vi "I2C Timestamp Loop.vi"(0 "fpga interface in":refnum<k20>, 1 "'stop' notifier":refnum<notifier>, 2 "log i2c to disk":bool=TRUE, 5 "tdms file directory":path, 9 "timestamp filter":T1[](array[typedef])=[enum."User24", enum."User25", enum."User26", enum."User27", enum."User28", enum."User29", enum."User30", enum."User31"], 11 "error in (no error)":errorcluster) -> (4 "i2c data":string[][](array[string]), 15 "error out":errorcluster)   [LabVIEW 2023, in "GettingStarted_Common_148X_Host.lvlib"]
uses:
  GettingStarted_Common_148X_Host.lvlib
  <instrlib>/FlexRIO/CSI-2/v2/FPGA/Types/Timestamp ID.ctl
  <instrlib>/FlexRIO/CSI-2/v2/FPGA/NI CSI-2 API FPGA v2.lvlib
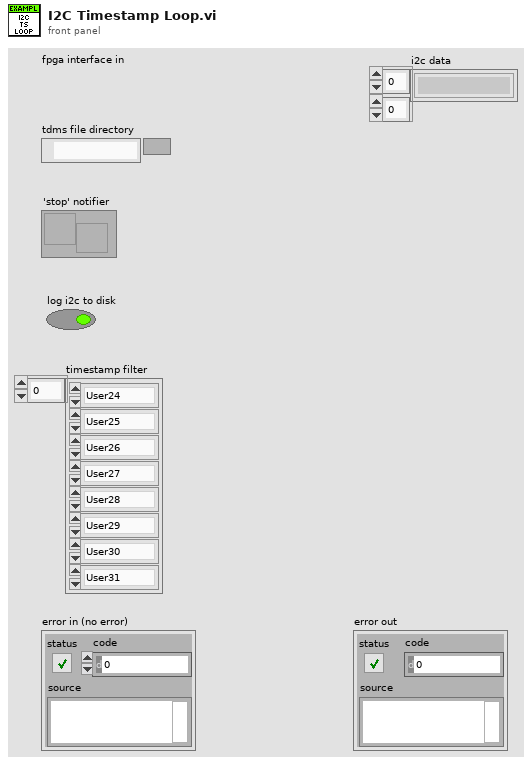
[diagram p1: front panel]
types:
  T1 = typedef "NI CSI-2 API FPGA v2.lvlib/Timestamp ID.ctl" = enum8{"SI0 LLP", "SI1 LLP", "SI2 LLP", "SI3 LLP", "SI4 LLP", "SI5 LLP", "SI6 LLP", "SI7 LLP", "SO0 LLP", "SO1 LLP", "SO2 LLP", "SO3 LLP", "SO4 LLP", "SO5 LLP", "SO6 LLP", "SO7 LLP", "Ser0 GPIO Bank", "Ser1 GPIO Bank", "Ser2 GPIO Bank", "Ser3 GPIO Bank", "Ser4 GPIO Bank", "Ser5 GPIO Bank", "Ser6 GPIO Bank", "Ser7 GPIO Bank", "Des0 GPIO Bank", "Des1 GPIO Bank", "Des2 GPIO Bank", "Des3 GPIO Bank", "Des4 GPIO Bank", "Des5 GPIO Bank", "Des6 GPIO Bank", "Des7 GPIO Bank", "User0", "User1", "User2", "User3", "User4", "User5", "User6", "User7", "User8", "User9", "User10", "User11", "User12", "User13", "User14", "User15", "User16", "User17", "User18", "User19", "User20", "User21", "User22", "User23", "User24", "User25", "User26", "User27", "User28", "User29", "User30", "User31"}
  T2 = typedef "NI CSI-2 API FPGA v2.lvlib/User Timestamp.ctl" = cluster{"valid":bool, "user data":fxp<+,58,58>, "id":T1}
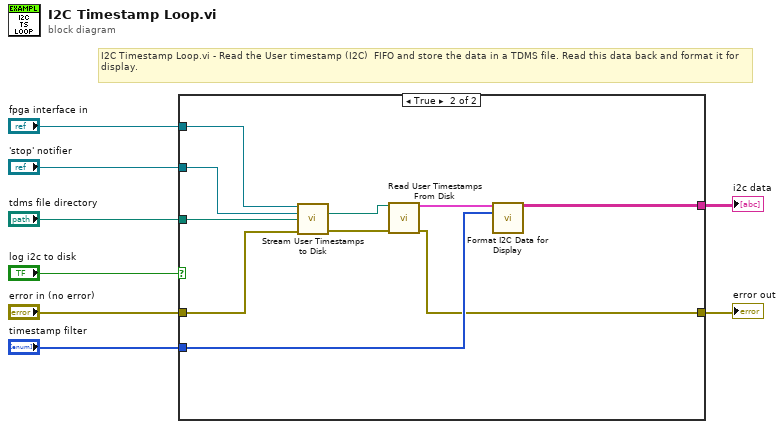
[diagram p0: block diagram]
diagram:
  # "I2C Timestamp Loop.vi - Read the User timestamp (I2C)  FIFO and store the data in a TDMS file. Read this data back and format it for display."
  n1 = case shown="True" "log i2c to disk" {
    tunnel: "error in (no error)" -> [w9 w19]
    tunnel: "fpga interface in" -> [_ w18]
    tunnel: "'stop' notifier" -> [_ w17]
    tunnel: "tdms file directory" -> [_ w16]
    tunnel: "timestamp filter" -> [_ w11]
    tunnel: [_ w12] -> w3
    tunnel: [w9 w10] -> w2
    frame False {
    }
    frame True {
      n2 = call "Stream User Timestamps to Disk.vi"("fpga interface in"=w18, "'stop' notifier"=w17, "base tdms file path"=w16, "error in (no error)"=w19) -> ("file path out"=w15:path, "error out"=w14:errorcluster)  [unwired: 8 in, 2 out]
      n3 = call "Read User Timestamps From Disk.vi"("file path"=w15, "error in (no error)"=w14) -> ("user timestamps"=w13:T2[], "error out"=w10:errorcluster)  [unwired: 12 in]
      n4 = call "Format I2C Data for Display.vi"("user timestamps"=w13, "timestamp filter"=w11) -> ("display data"=w12:string[][])  [unwired: 13 in]
    }
  }
  "error out" <- w2
  "i2c data" <- w3
